vi "_Calculate cps.vi"(1 "Dwell (mS)":dbl, 2 "Raw Counts":i32[](array[numeric])) -> (0 "Data in cps":dbl[](array[numeric]))   [LabVIEW 2015]
uses:
  _Global Configuration.vi
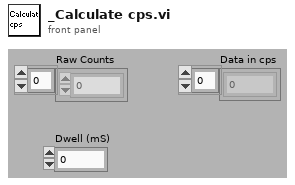
[diagram p1: front panel]
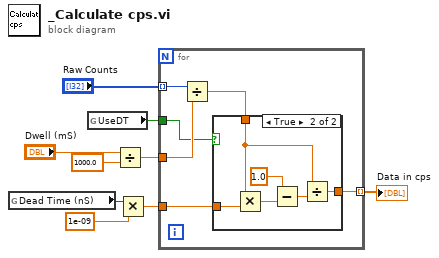
[diagram p0: block diagram]
diagram:
  n1 = global read "_Global Configuration.vi" "Dead Time (nS)"() -> (w6:i32)
  n2 = global read "_Global Configuration.vi" "UseDT"() -> (w2:bool)
  n3 = Divide(x="Dwell (mS)", y=1000.0) -> (x/y=w9:dbl)
  n4 = Multiply(x=w6, y=1e-09) -> (x*y=w4:dbl)
  n5 = for {
    tunnel: w9 -> [w15]
    tunnel: "Raw Counts" -> [w14] mode=indexing
    tunnel: w4 -> [w13]
    tunnel: [w11] -> w3 mode=indexing
    tunnel: w2 -> [w10]
    n6 = Divide(x=w14, y=w15) -> (x/y=w12:dbl)
    n7 = case shown="True" w10 {
      tunnel: w13 -> [_ w22]
      tunnel: w12 -> [w16 w18]
      tunnel: [w16 w17] -> w11
      frame False {
      }
      frame True {
        n8 = Multiply(x=w18, y=w22) -> (x*y=w21:dbl)
        n9 = Subtract(x=1.0 ("y"), y=w21) -> (x-y=w19:dbl)
        n10 = Divide(x=w18, y=w19) -> (x/y=w17:dbl)
      }
    }
  }
  "Data in cps" <- w3
